vi "Create Action Queue.vi"(11 "error in":errorcluster) -> (4 "action queue out":refnum<queue>, 15 "error out":errorcluster)   [LabVIEW 2016, in "TLB` Template.lvlib" / "Actions.lvlib"]
doc: "Create action queue resource for communication.\n\n<B>Input Parameters</B>\n\n<B>error in</B> describes error conditions that occur before this node runs. This input provides standard error in functionality.\n\n<B>Output Parameters</B>\n\n<B>action queue out</B> is a reference to the existing queue or the new queue created by this function.\n\n<B>error out</B> contains error information. This output provides standard error out functionality."
uses:
  Actions.lvlib
  System Action Element.ctl
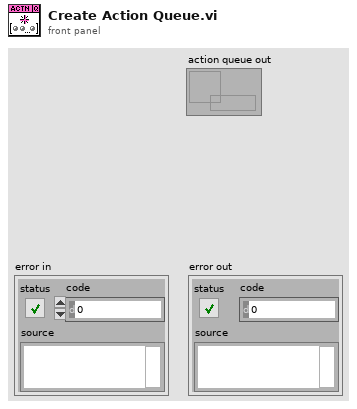
[diagram p1: front panel]
types:
  T1 = typedef "TLB` Template.lvlib/Actions.lvlib/System Action Element.ctl" = cluster{"action":string, "data":string}
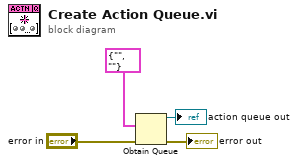
[diagram p0: block diagram]
diagram:
  n1 = Obtain Queue(element data type=T1 {"action"="", "data"=""}, error in (no error)="error in") -> (queue out=→"action queue out":refnum<queue>, error out=→"error out":errorcluster)  [unwired: 3 in, 1 out]
